vi "Set Class CSV_File.vi"(8 "error in (no error)":errorcluster caption="entrée d'erreur (pas d'erreur)", 10 "Library File.lvlib:Class CSV_File.lvclass":refnum<class "Class CSV_File.lvclass">, 11 "Class Log_File (Default) en entrée":refnum<class "Class Log_File (Default).lvclass">) -> (0 "error out":errorcluster caption="sortie d'erreur", 3 "Class Log_File (Default) en sortie":refnum<class "Class Log_File (Default).lvclass">)   [LabVIEW 2020, in "Library Instrument & Equipement.lvlib" / "Library Log_File.lvlib" / "Class Log_File (Default).lvclass"]
uses:
  Class Log_File (Default).lvclass
  Read CSV File/CSV_File (Default)/Class CSV_File.lvclass
  Class Log_File (Default).lvclass/Class Log_File (Default).ctl
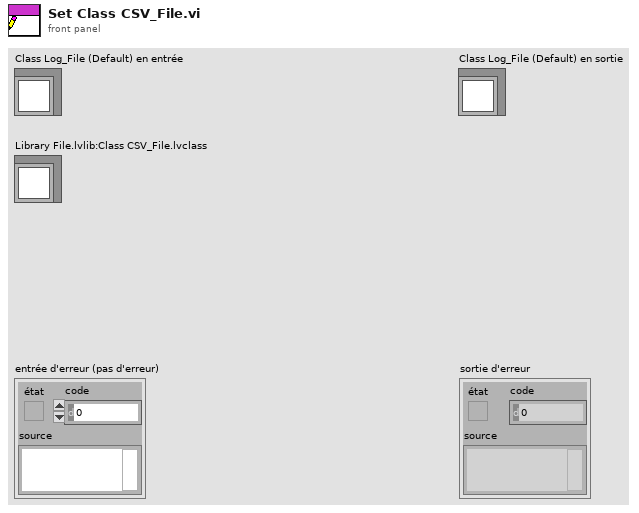
[diagram p1: front panel]
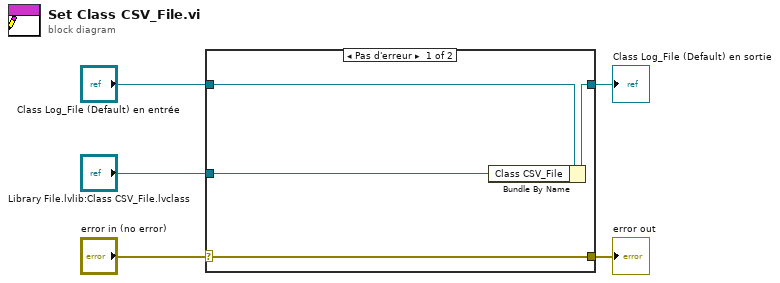
[diagram p0: block diagram]
diagram:
  n1 = case shown="Pas d'erreur" "error in (no error)" {
    selector: "error in (no error)" -> [w9 w10]
    tunnel: [w9 w10] -> w4
    tunnel: [w7 w11] -> w2
    tunnel: "Class Log_File (Default) en entrée" -> [w8 w11]
    tunnel: "Library File.lvlib:Class CSV_File.lvclass" -> [w6 _]
    frame No Error {
      n2 = Bundle By Name(cluster=w8, "Class CSV_File"=w6) -> (w7:refnum<class "Class Log_File (Default).lvclass">)
    }
    frame Error {
    }
  }
  "error out" <- w4
  "Class Log_File (Default) en sortie" <- w2
